vi "Omni-Driver-Fast-Close.vi"(1 "Wrapper In":u32) -> ()   [LabVIEW 2014]
doc: "André Romero - 2017\nandretec@ifsc.usp.br"
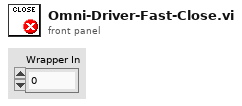
[diagram p1: front panel]
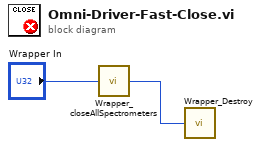
[diagram p0: block diagram]
diagram:
  n1 = call "Wrapper_closeAllSpectrometers.vi"("Wrapper In"="Wrapper In") -> ("Wrapper Out"=w2:u32)
  n2 = call "Wrapper_Destroy.vi"("Wrapper"=w2) -> ()
